vi "RT.Stages.Find.vi"(8 "Current Data":dbl[](array[numeric]), 9 "Voltage Data":dbl[](array[numeric]), 10 "Shots":T1[](array[typedef]) {"Results"."Off-Stage Min Volt" format="%#.6g"; "Results"."Off-Stage Avg Volt" format="%#.6g"; "Results"."Off-Stage Max Volt" format="%#.6g"; "Results"."Total Stage Time (us)" format="%#.6g"; "Results"."Off-Stage Avg Current" format="%#.6g"; "Results"."Total Voltage Pulses" format="%#.6g"; "Results"."Off-Stage Min Current" format="%#.6g"; "Results"."Off-Stage Max Current" format="%#.6g"}, 11 "Parameters":T3={"Shots"=0, "Shot.InitialVoltage"=0.0, "Shot.Stages"=0, "Stages"=[{"Stage.Dwell.Level"=0.0, "PullIn.Type"=enum."Pull In Transition Pulses", "PullIn.Level"=0.0, "Transition.Type"=enum."Stage Transition Voltage Increase", "Transition.Level"=0.0, "Results"={"Pull In Time"=TRUE, "Pull In Max Current"=TRUE, "Pull In Max Voltage"=TRUE, "Pull In Min Voltage"=TRUE, "Pull In Avg Voltage"=TRUE, "Hold Time"=TRUE, "Hold Max Current"=TRUE, "Hold Min Current"=TRUE, "Hold Avg Current"=TRUE, "Hold Max Voltage"=TRUE, "Hold Min Voltage"=TRUE, "Hold Avg Max Voltage"=TRUE, "Hold Avg Min Voltage"=TRUE, "Off Time"=TRUE, "Off Max Current"=TRUE, "Off Min Current"=TRUE, "Off Avg Current"=TRUE, "Off Max Voltage"=TRUE, "Off Min Voltage"=TRUE, "Off Avg Voltage"=TRUE, "Total Voltage Pulses"=TRUE, "Total Stage Time"=TRUE}}], "Timeout"=0.0, "Results.Count"=0, "Active Edge"=FALSE, "Rate.Hz"=0, "Channels"=0}) -> (2 "Shots":T1[](array[typedef]) {"Results"."Off-Stage Min Volt" format="%#.6g"; "Results"."Off-Stage Avg Volt" format="%#.6g"; "Results"."Off-Stage Max Volt" format="%#.6g"; "Results"."Total Stage Time (us)" format="%#.6g"; "Results"."Off-Stage Avg Current" format="%#.6g"; "Results"."Total Voltage Pulses" format="%#.6g"; "Results"."Off-Stage Min Current" format="%#.6g"; "Results"."Off-Stage Max Current" format="%#.6g"})   [LabVIEW 2019, in "Fuel Injector Analysis Addon Engine.lvlib"]
uses:
  Fuel Injector Analysis Addon Engine.lvlib
  Addon Shared/Types/Shot.Parameters.ctl
  Addon Shared/Types/Stage.Parameters.ctl
  Addon Shared/Types/Stage.PullIn.Types.ctl
  Addon Shared/Types/Stage.Transition.Types.ctl
  Addon Shared/Types/Analysis.Channels.Select.ctl
  RT Analysis/Controls/Shot Information Control.ctl
  Types/Stage.Measurements.ctl
  Types/Search.StateVariables.ctl
  Addon Shared/Types/Stage.Events.ctl
  Addon Shared/Fuel Injector Analysis Addon Shared.lvlib
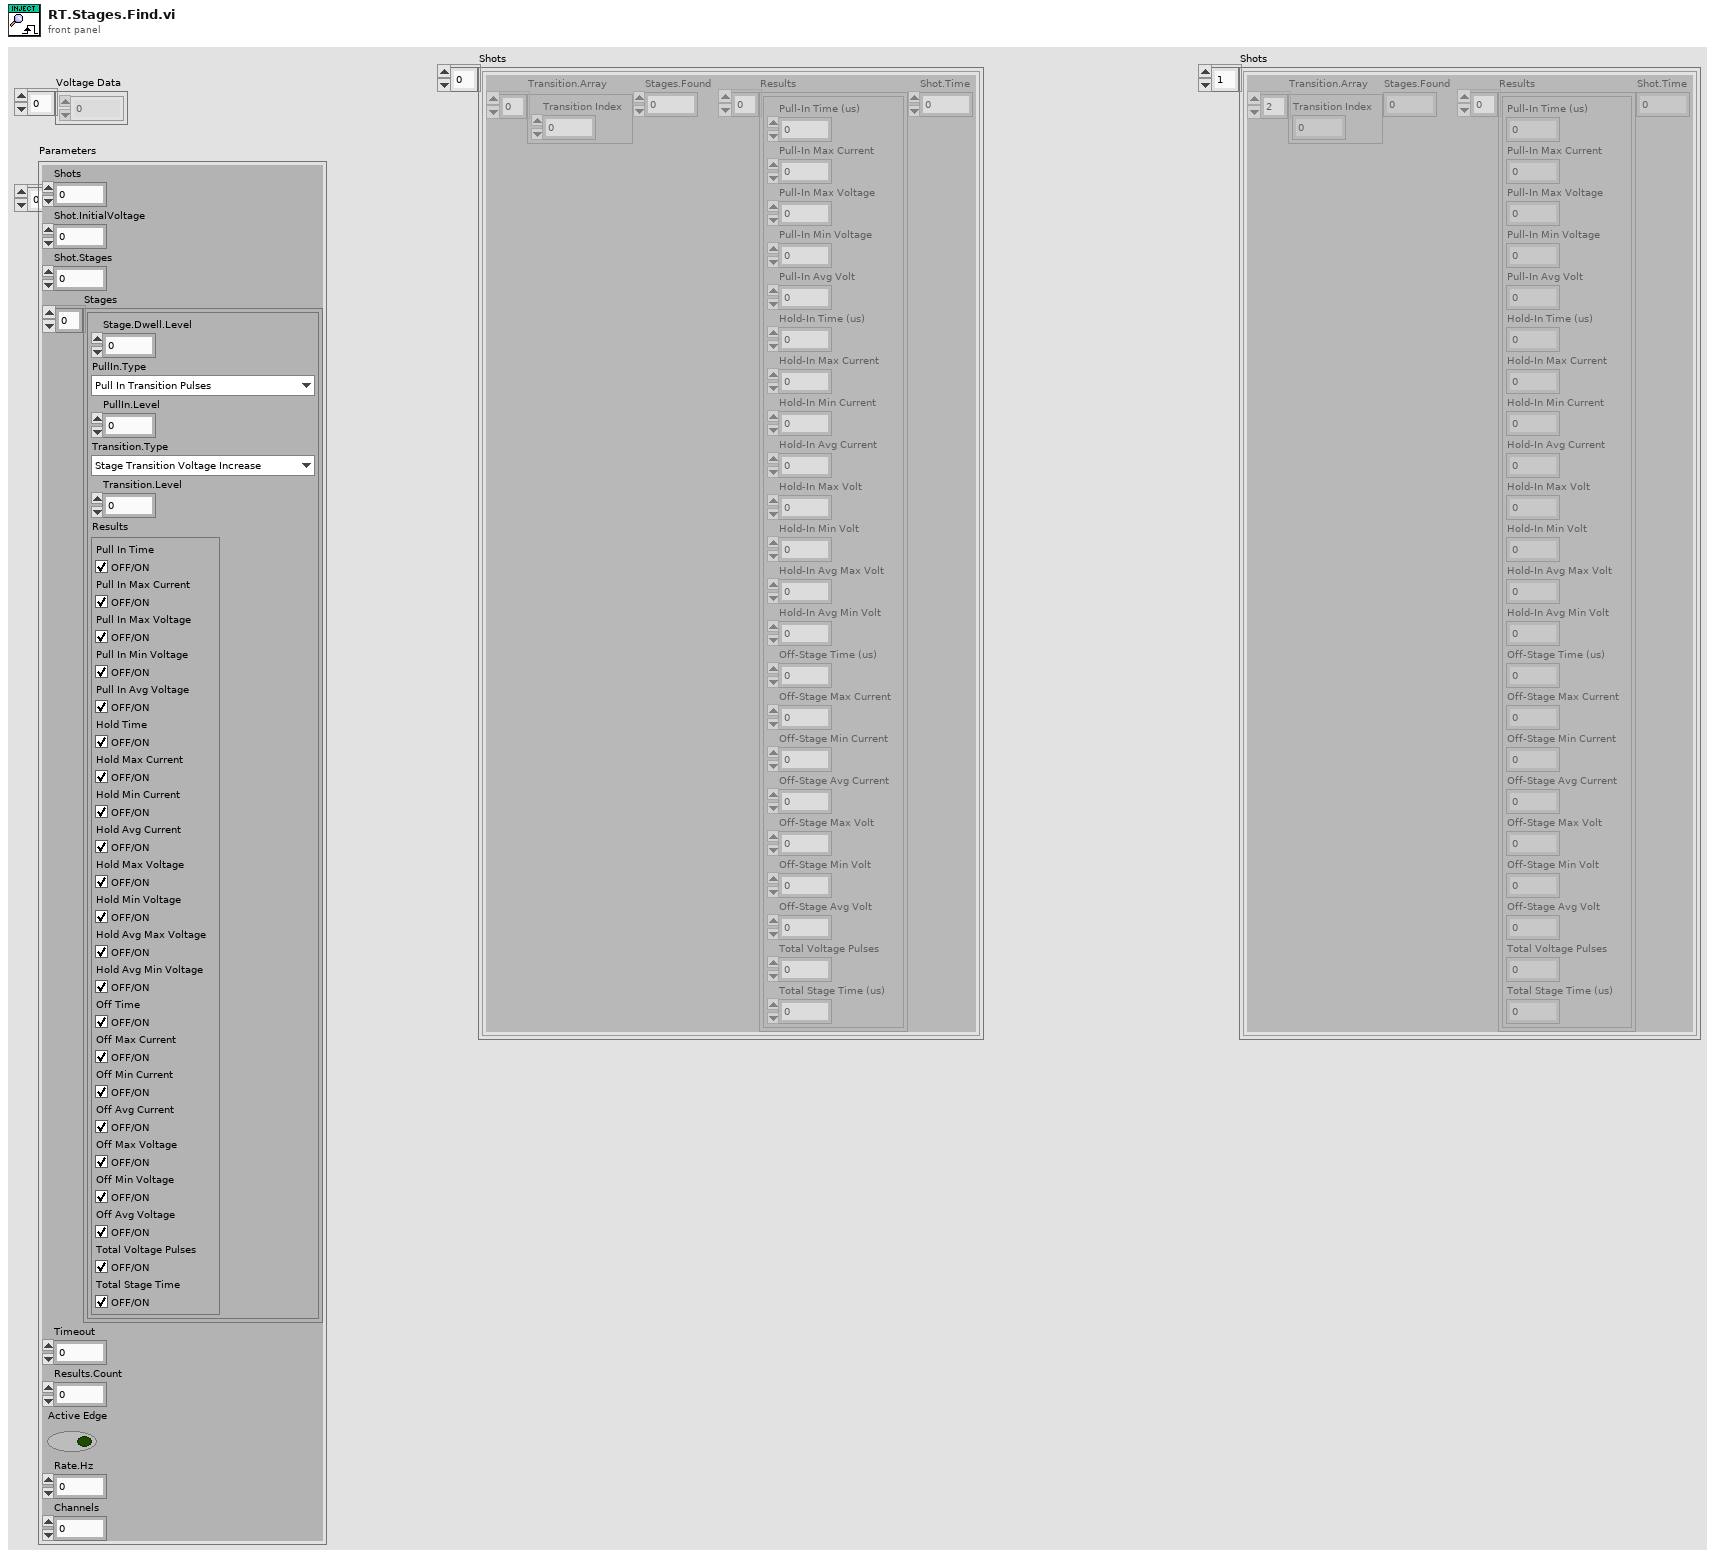
[diagram p1: front panel]
types:
  T1 = typedef "Fuel Injector Analysis Addon Engine.lvlib/Shot Information Control.ctl" = cluster{"Transition.Array":i32[], "Stages.Found":u16, "Results":T2[], "Shot.Time":dbl}
  T2 = typedef "Fuel Injector Analysis Addon Engine.lvlib/Stage.Measurements.ctl" = cluster{"Pull-In Time (us)":dbl, "Pull-In Max Current":dbl, "Pull-In Max Voltage":dbl, "Pull-In Min Voltage":dbl, "Pull-In Avg Volt":dbl, "Hold-In Time (us)":dbl, "Hold-In Max Current":dbl, "Hold-In Min Current":dbl, "Hold-In Avg Current":dbl, "Hold-In Max Volt":dbl, "Hold-In Min Volt":dbl, "Hold-In Avg Max Volt":dbl, "Hold-In Avg Min Volt":dbl, "Off-Stage Time (us)":dbl, "Off-Stage Max Current":dbl, "Off-Stage Min Current":dbl, "Off-Stage Avg Current":dbl, "Off-Stage Max Volt":dbl, "Off-Stage Min Volt":dbl, "Off-Stage Avg Volt":dbl, "Total Voltage Pulses":dbl, "Total Stage Time (us)":dbl}
  T3 = typedef "Fuel Injector Analysis Addon Shared.lvlib/Shot.Parameters.ctl" = cluster{"Shots":u32, "Shot.InitialVoltage":dbl, "Shot.Stages":u32, "Stages":T4[], "Timeout":dbl, "Results.Count":i32, "Active Edge":bool, "Rate.Hz":u32, "Channels":u32}
  T4 = typedef "Fuel Injector Analysis Addon Shared.lvlib/Stage.Parameters.ctl" = cluster{"Stage.Dwell.Level":dbl, "PullIn.Type":T5, "PullIn.Level":dbl, "Transition.Type":T6, "Transition.Level":dbl, "Results":T7}
  T5 = typedef "Fuel Injector Analysis Addon Shared.lvlib/Stage.PullIn.Types.ctl" = enum8{"Pull In Transition Pulses", "Pull In Transition Current Drop"}
  T6 = typedef "Fuel Injector Analysis Addon Shared.lvlib/Stage.Transition.Types.ctl" = enum8{"Stage Transition Inactive Time", "Stage Transition Voltage Increase", "Stage Transition Current Decrease", "Stage Transition Active Time"}
  T7 = typedef "Fuel Injector Analysis Addon Shared.lvlib/Analysis.Channels.Select.ctl" = cluster{"Pull In Time":bool, "Pull In Max Current":bool, "Pull In Max Voltage":bool, "Pull In Min Voltage":bool, "Pull In Avg Voltage":bool, "Hold Time":bool, "Hold Max Current":bool, "Hold Min Current":bool, "Hold Avg Current":bool, "Hold Max Voltage":bool, "Hold Min Voltage":bool, "Hold Avg Max Voltage":bool, "Hold Avg Min Voltage":bool, "Off Time":bool, "Off Max Current":bool, "Off Min Current":bool, "Off Avg Current":bool, "Off Max Voltage":bool, "Off Min Voltage":bool, "Off Avg Voltage":bool, "Total Voltage Pulses":bool, "Total Stage Time":bool}
  T8 = typedef "Fuel Injector Analysis Addon Engine.lvlib/Search.StateVariables.ctl" = cluster{"Dwell.Counts":i32, "Current.Max":dbl, "Stage.Index":i32, "Transition.Index":i32, "Transition":T9}
  T9 = typedef "Fuel Injector Analysis Addon Shared.lvlib/Stage.Events.ctl" = enum8{"PullIn.Start", "PullIn.End", "Dwell.End"}
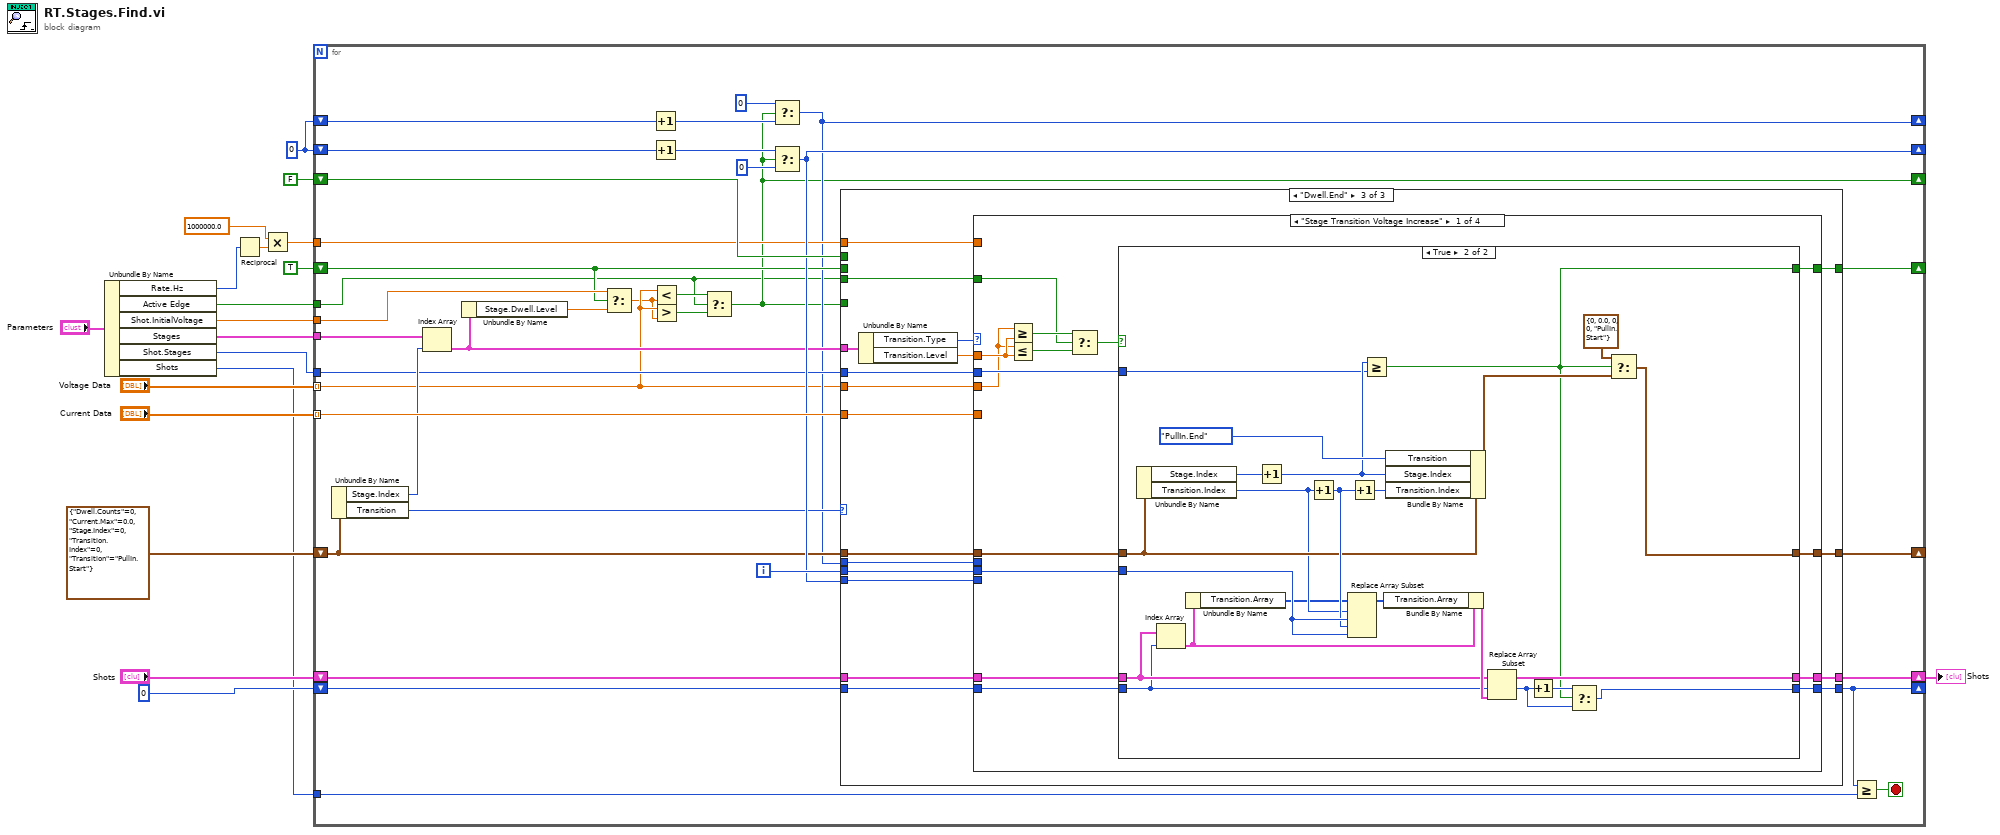
[diagram p0: block diagram]
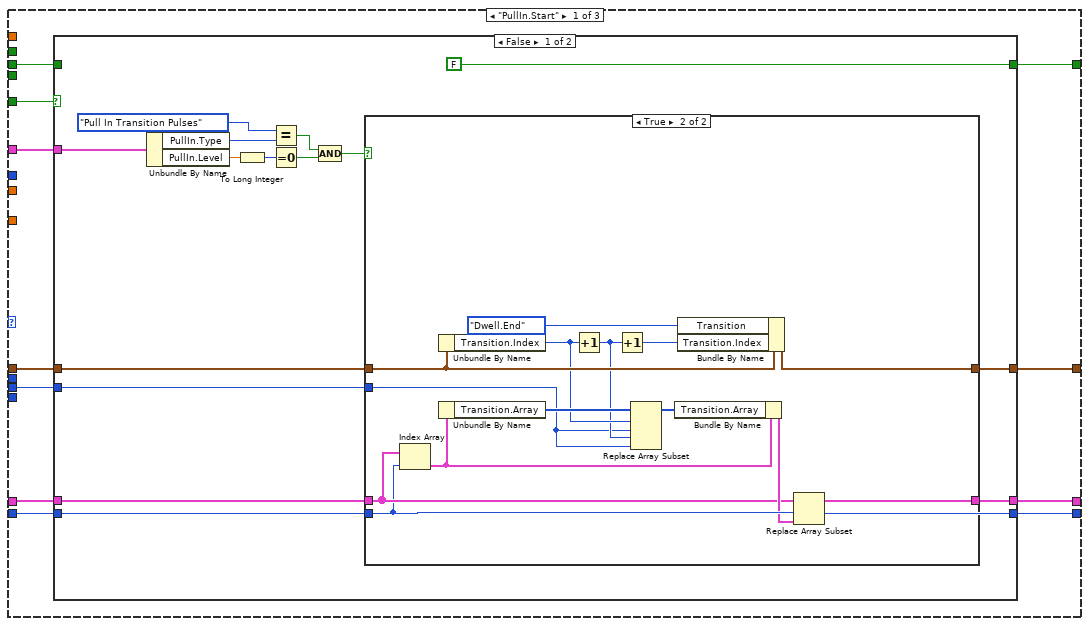
[diagram p2: hidden frame]
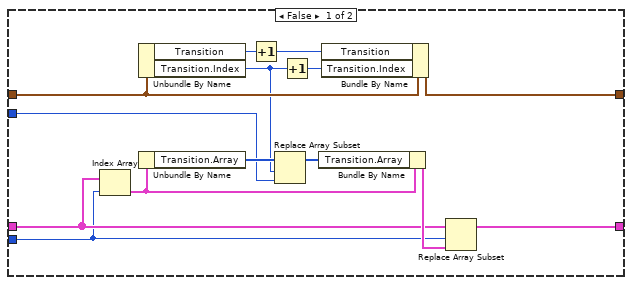
[diagram p3: hidden frame]
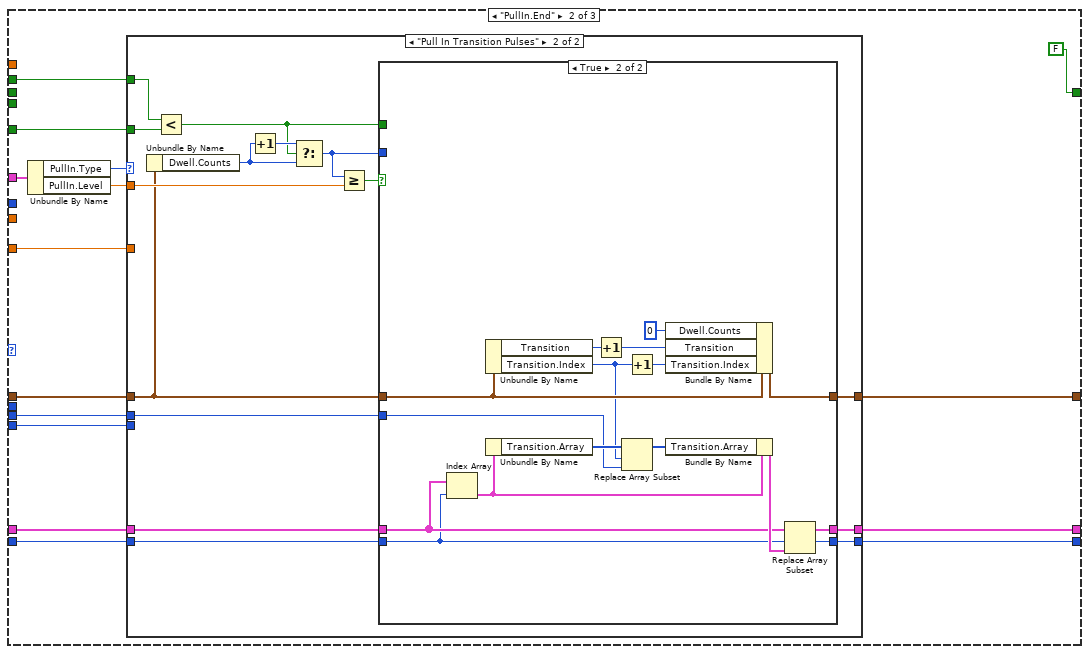
[diagram p5: hidden frame]
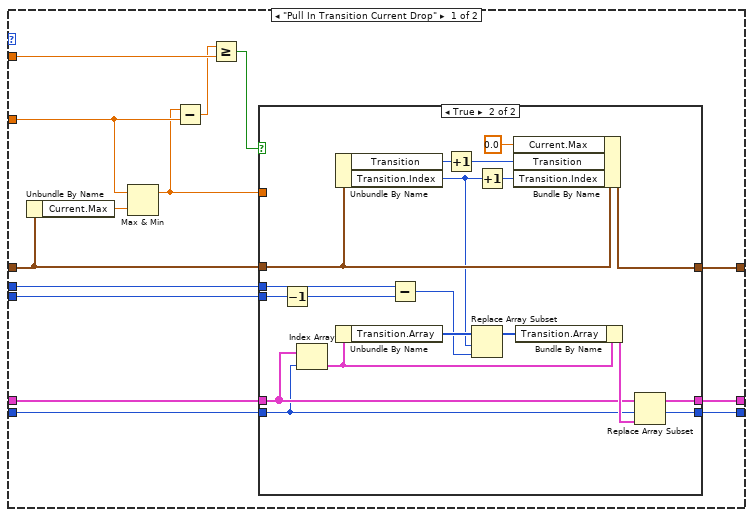
[diagram p6: hidden frame]
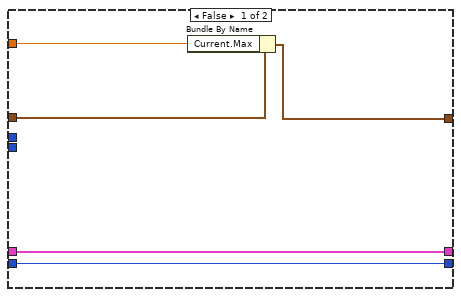
[diagram p7: hidden frame]
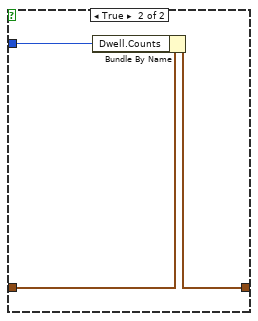
[diagram p9: hidden frame]
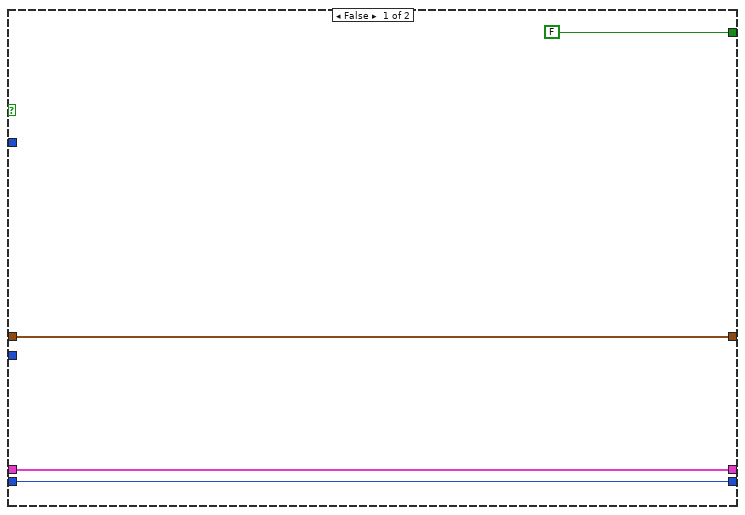
[diagram p10: hidden frame]
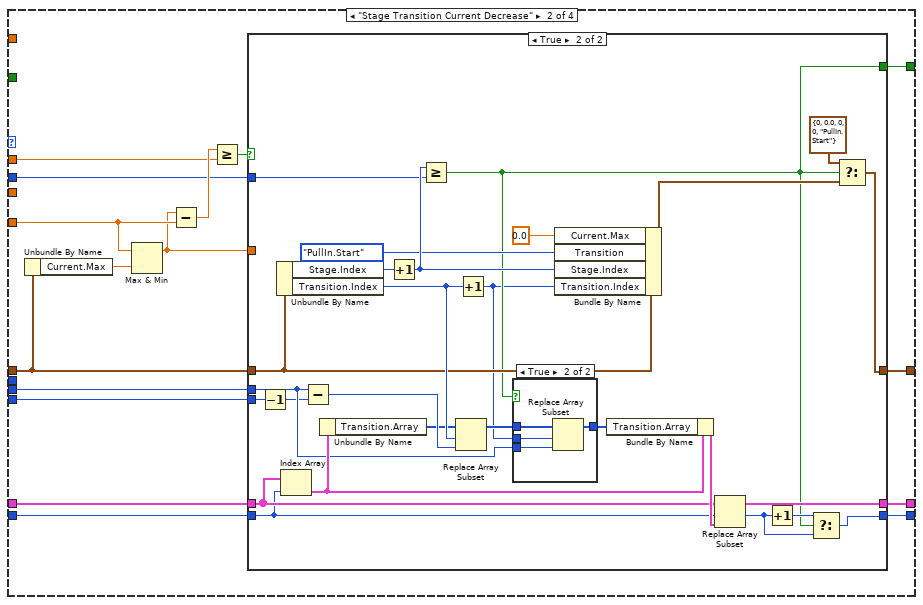
[diagram p11: hidden frame]
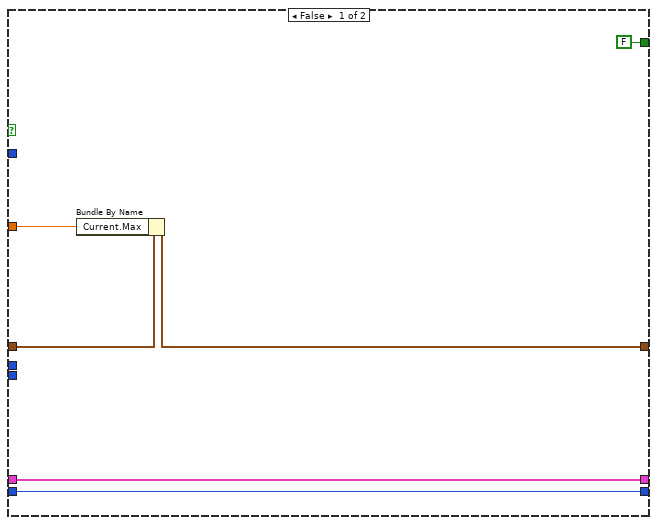
[diagram p12: hidden frame]
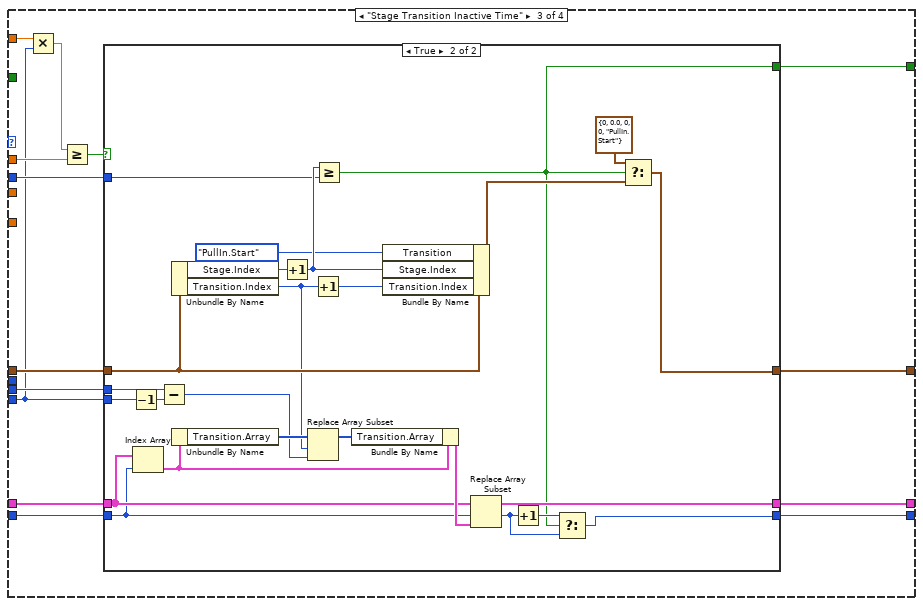
[diagram p14: hidden frame]
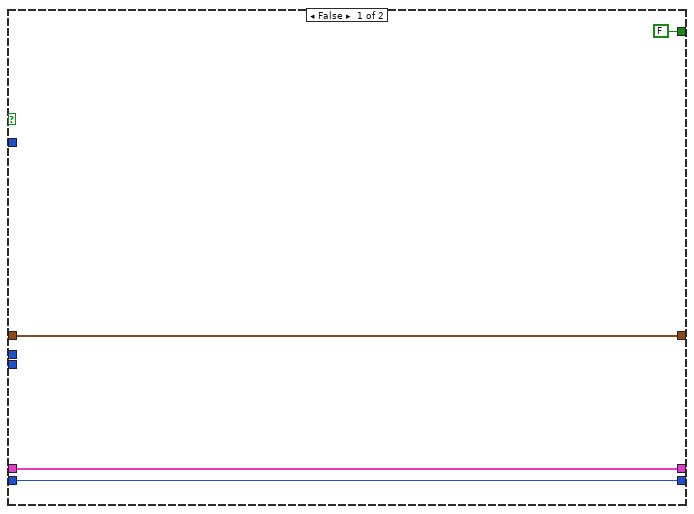
[diagram p15: hidden frame]
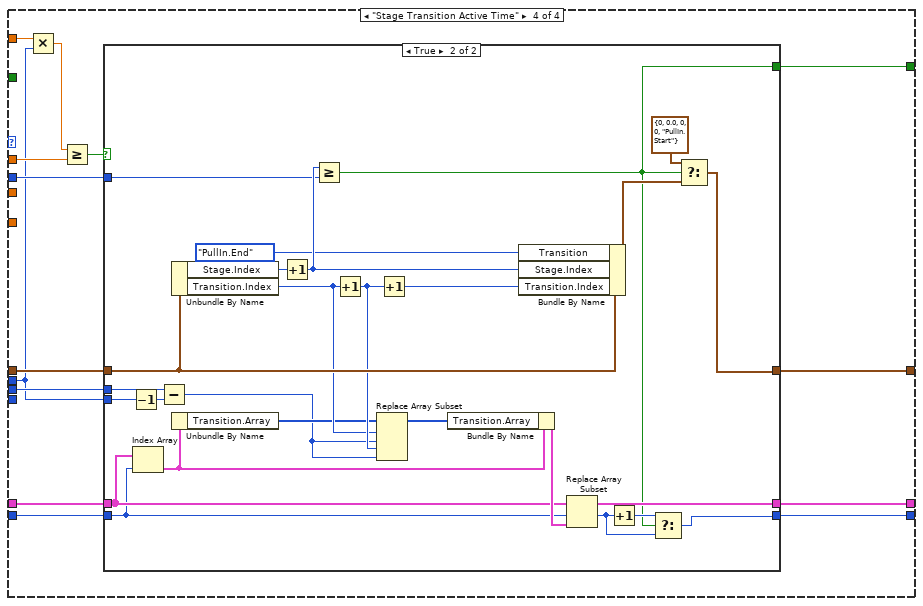
[diagram p16: hidden frame]
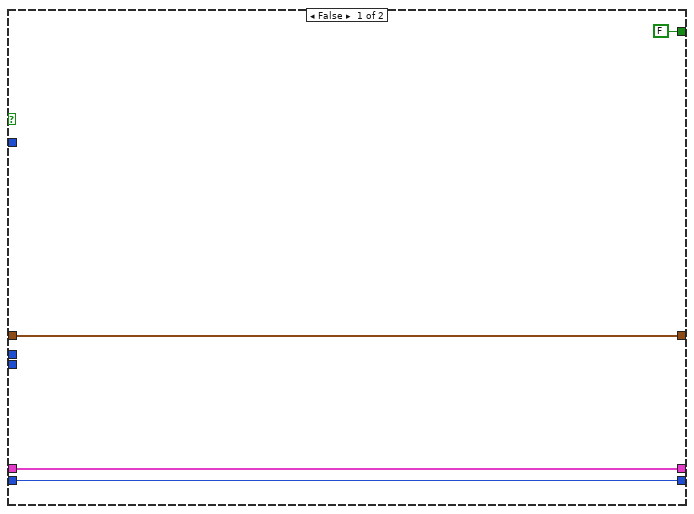
[diagram p17: hidden frame]
diagram:
  w3 = 0
  n1 = Unbundle By Name("Parameters") -> ("Rate.Hz"=w1:u32, "Active Edge"=w2:bool, "Shot.InitialVoltage"=w14:dbl, "Stages"=w15:T4[], "Shot.Stages"=w10:u32, "Shots"=w8:u32)
  n2 = Reciprocal(x=w1) -> (1/x=w6:dbl)
  n3 = Multiply(x=1000000.0, y=w6) -> (x*y=w5:dbl)
  n4 = for {
    tunnel: "Voltage Data" -> [w25] mode=indexing
    tunnel: "Current Data" -> [w53] mode=indexing
    tunnel: w15 -> [w54]
    shift-right: [w21] -> _
    shift-left: FALSE -> [w48]
    shift-right: [w47] -> _
    shift-left: w3 -> [w49]
    shift-right: [w42] -> _
    shift-left: T8 {"Dwell.Counts"=0, "Current.Max"=0.0, "Stage.Index"=0, "Transition.Index"=0, "Transition"=enum."PullIn.Start"} -> [w43]
    tunnel: w14 -> [w34]
    shift-right: [w40] -> w12
    shift-left: "Shots" -> [w41]
    shift-right: [w37] -> _
    shift-left: 0 -> [w39]
    tunnel: w10 -> [w38]
    tunnel: w8 -> [w36]
    shift-right: [w32] -> _
    shift-left: TRUE -> [w31]
    tunnel: w5 -> [w30]
    shift-right: [w26] -> _
    shift-left: w3 -> [w29]
    tunnel: w2 -> [w20]
    i -> [w52]
    stop <- w35 stop-if-true
    n5 = Unbundle By Name(w43) -> ("Stage.Index"=w44:i32, "Transition"=w45:T9)
    n6 = Index Array(array=w54, index=w44) -> (element=w46:T4)
    n7 = Unbundle By Name(w46) -> ("Stage.Dwell.Level"=w33:dbl)
    n8 = Select(t=w34, s=w31, f=w33) -> (s? t:f=w24:dbl)
    n9 = Increment(x=w29) -> (x+1=w28:i32)
    n10 = Increment(x=w49) -> (x+1=w51:i32)
    n11 = Less?(x=w25, y=w24) -> (x < y?=w22:bool)
    n12 = Greater?(x=w25, y=w24) -> (0:w23:bool)
    n13 = Select(t=w22, s=w20, f=w23) -> (s? t:f=w21:bool)
    n14 = Select(t=0 ("f"), s=w21, f=w28) -> (s? t:f=w26:i32)
    n15 = Select(t=w51, s=w21, f=0) -> (s? t:f=w47:i32)
    n16 = case shown="\"Dwell.End\"" w45 {
      tunnel: w53 -> [_ w127 w216]
      tunnel: w25 -> [_ _ w222]
      tunnel: w52 -> [w65 w124 w221]
      tunnel: w48 -> [_ w120 _]
      tunnel: w21 -> [w58 w121 _]
      tunnel: w47 -> [_ w123 w220]
      tunnel: w46 -> [w55 w126 w219]
      tunnel: w43 -> [w64 w119 w215]
      tunnel: [w63 w118 w214] -> w42
      tunnel: w41 -> [w62 w117 w213]
      tunnel: [w61 w114 w212] -> w40
      tunnel: w39 -> [w60 w116 w211]
      tunnel: [w59 w115 w210] -> w37
      tunnel: w38 -> [_ _ w209]
      tunnel: [w57 FALSE w208] -> w32
      tunnel: w31 -> [w56 _ _]
      tunnel: w30 -> [_ _ w207]
      tunnel: w26 -> [_ _ w206]
      tunnel: w20 -> [_ _ w205]
      frame "PullIn.Start" {
        n17 = case shown="False" w58 {
          tunnel: w65 -> [w76 _]
          tunnel: w64 -> [w80 w112]
          tunnel: [w79 w112] -> w63
          tunnel: w62 -> [w78 w111]
          tunnel: [w77 w111] -> w61
          tunnel: w60 -> [w75 w110]
          tunnel: [w75 w110] -> w59
          tunnel: [FALSE w109] -> w57
          tunnel: w56 -> [_ w109]
          tunnel: w55 -> [w73 _]
          frame False {
            n18 = Unbundle By Name(w73) -> ("PullIn.Type"=w72:T5, "PullIn.Level"=w70:dbl)
            n19 = To Long Integer(number=w70) -> (32bit integer=w69:i32)
            n20 = Equal?(x=Stage.PullIn.Types."Pull In Transition Pulses", y=w72) -> (x = y?=w68:bool)
            n21 = Equal To 0?(x=w69) -> (x = 0?=w67:bool)
            n22 = Compound Arithmetic op=AND(w68, w67) -> (w66:bool)
            n23 = case shown="True" w66 {
              tunnel: w80 -> [w93 w108]
              tunnel: [w90 w107] -> w79
              tunnel: w78 -> [w85 w102]
              tunnel: [w84 w101] -> w77
              tunnel: w76 -> [w83 w95]
              tunnel: w75 -> [w81 w99]
              frame False {
                n24 = Index Array(array=w85, index=w81) -> (element=w87:T1)
                n25 = Unbundle By Name(w93) -> ("Transition"=w94:T9, "Transition.Index"=w82:i32)
                n26 = Unbundle By Name(w87) -> ("Transition.Array"=w86:i32[])
                n27 = Increment(x=w94) -> (x+1=w91:T9)
                n28 = Replace Array Subset(array=w86, new element=w83, index=w82) -> (w89:i32[])
                n29 = Increment(x=w82) -> (x+1=w92:i32)
                n30 = Bundle By Name(cluster=w87, "Transition.Array"=w89) -> (w88:T1)
                n31 = Bundle By Name(cluster=w93, "Transition"=w91, "Transition.Index"=w92) -> (w90:T8)
                n32 = Replace Array Subset(array=w85, new element=w88, index=w81) -> (w84:T1[])
              }
              frame True {
                n33 = Index Array(array=w102, index=w99) -> (element=w104:T1)
                n34 = Unbundle By Name(w108) -> ("Transition.Index"=w100:i32)
                n35 = Unbundle By Name(w104) -> ("Transition.Array"=w103:i32[])
                n36 = Increment(x=w100) -> (x+1=w96:i32)
                n37 = Increment(x=w96) -> (x+1=w97:i32)
                n38 = Replace Array Subset(array=w103, new element #1=w95, index #1=w100, new element #2=w95, index #2=w96) -> (w106:i32[])
                n39 = Bundle By Name(cluster=w104, "Transition.Array"=w106) -> (w105:T1)
                n40 = Bundle By Name(cluster=w108, "Transition"=Stage.Events."Dwell.End", "Transition.Index"=w97) -> (w107:T8)
                n41 = Replace Array Subset(array=w102, new element=w105, index=w99) -> (w101:T1[])
              }
            }
          }
          frame True {
          }
        }
      }
      frame "PullIn.End" {
        n42 = Unbundle By Name(w126) -> ("PullIn.Type"=w122:T5, "PullIn.Level"=w125:dbl)
        n43 = case shown="\"Pull In Transition Pulses\"" w122 {
          tunnel: w127 -> [w141 _]
          tunnel: w125 -> [w140 w179]
          tunnel: w124 -> [w138 w173]
          tunnel: w123 -> [w137 _]
          tunnel: w121 -> [_ w176]
          tunnel: w120 -> [_ w175]
          tunnel: w119 -> [w134 w172]
          tunnel: [w132 w174] -> w118
          tunnel: w117 -> [w131 w168]
          tunnel: w116 -> [w130 w167]
          tunnel: [w129 w166] -> w115
          tunnel: [w128 w165] -> w114
          frame "Pull In Transition Current Drop" {
            n44 = Unbundle By Name(w134) -> ("Current.Max"=w135:dbl)
            n45 = Max & Min(x=w141, y=w135) -> (max(x,y)=w133:dbl)  [unwired: 1 out]
            n46 = Subtract(x=w133, y=w141) -> (x-y=w136:dbl)
            n47 = Greater Or Equal?(x=w136, y=w140) -> (x >= y?=w139:bool)
            n48 = case shown="True" w139 {
              tunnel: w138 -> [_ w164]
              tunnel: w137 -> [_ w163]
              tunnel: w134 -> [w146 w157]
              tunnel: w133 -> [w145 _]
              tunnel: [w144 w158] -> w132
              tunnel: w131 -> [w142 w152]
              tunnel: w130 -> [w143 w149]
              tunnel: [w143 w149] -> w129
              tunnel: [w142 w148] -> w128
              frame False {
                n49 = Bundle By Name(cluster=w146, "Current.Max"=w145) -> (w144:T8)
              }
              frame True {
                n50 = Decrement(x=w163) -> (x-1=w147:i32)
                n51 = Index Array(array=w152, index=w149) -> (element=w154:T1)
                n52 = Unbundle By Name(w157) -> ("Transition"=w159:T9, "Transition.Index"=w150:i32)
                n53 = Unbundle By Name(w154) -> ("Transition.Array"=w153:i32[])
                n54 = Subtract(x=w164, y=w147) -> (x-y=w151:i32)
                n55 = Increment(x=w159) -> (x+1=w161:T9)
                n56 = Replace Array Subset(array=w153, new element=w151, index=w150) -> (w156:i32[])
                n57 = Increment(x=w150) -> (x+1=w160:i32)
                n58 = Bundle By Name(cluster=w157, "Current.Max"=0.0 ("Dwell.Counts"), "Transition"=w161, "Transition.Index"=w160) -> (w158:T8)
                n59 = Bundle By Name(cluster=w154, "Transition.Array"=w156) -> (w155:T1)
                n60 = Replace Array Subset(array=w152, new element=w155, index=w149) -> (w148:T1[])
              }
            }
          }
          frame "Pull In Transition Pulses" {
            n61 = Unbundle By Name(w172) -> ("Dwell.Counts"=w171:i32)
            n62 = Less?(x=w175, y=w176) -> (x < y?=w169:bool)
            n63 = Increment(x=w171) -> (x+1=w177:i32)
            n64 = Select(t=w177, s=w169, f=w171) -> (s? t:f=w170:i32)
            n65 = Greater Or Equal?(x=w170, y=w179) -> (x >= y?=w178:bool)
            n66 = case shown="True" w178 {
              tunnel: w172 -> [w185 w201]
              tunnel: [w184 w200] -> w174
              tunnel: w173 -> [_ w192]
              tunnel: w170 -> [w183 _]
              tunnel: w169 -> [w182 _]
              tunnel: w168 -> [w180 w194]
              tunnel: w167 -> [w181 w193]
              tunnel: [w181 w193] -> w166
              tunnel: [w180 w190] -> w165
              frame False {
                n67 = case shown="False" w182 {
                  tunnel: w185 -> [w186 w189]
                  tunnel: [w186 w188] -> w184
                  tunnel: w183 -> [_ w187]
                  frame False {
                  }
                  frame True {
                    n68 = Bundle By Name(cluster=w189, "Dwell.Counts"=w187) -> (w188:T8)
                  }
                }
              }
              frame True {
                n69 = Index Array(array=w194, index=w193) -> (element=w196:T1)
                n70 = Unbundle By Name(w201) -> ("Transition"=w204:T9, "Transition.Index"=w191:i32)
                n71 = Unbundle By Name(w196) -> ("Transition.Array"=w195:i32[])
                n72 = Increment(x=w204) -> (x+1=w202:T9)
                n73 = Replace Array Subset(array=w195, new element=w192, index=w191) -> (w198:i32[])
                n74 = Increment(x=w191) -> (x+1=w203:i32)
                n75 = Bundle By Name(cluster=w201, "Dwell.Counts"=0, "Transition"=w202, "Transition.Index"=w203) -> (w200:T8)
                n76 = Bundle By Name(cluster=w196, "Transition.Array"=w198) -> (w197:T1)
                n77 = Replace Array Subset(array=w194, new element=w197, index=w193) -> (w190:T1[])
              }
            }
          }
        }
      }
      frame "Dwell.End" {
        n78 = Unbundle By Name(w219) -> ("Transition.Type"=w218:T6, "Transition.Level"=w217:dbl)
        n79 = case shown="\"Stage Transition Voltage Increase\"" w218 {
          tunnel: w222 -> [w227 _ _ _]
          tunnel: w221 -> [w237 w275 w327 w369]
          tunnel: w217 -> [w228 w277 w329 w371]
          tunnel: w220 -> [_ w274 w319 _]
          tunnel: w216 -> [_ w278 _ _]
          tunnel: w215 -> [w236 w273 w328 w370]
          tunnel: [w235 w271 w326 w368] -> w214
          tunnel: w213 -> [w234 w269 w325 w367]
          tunnel: [w233 w268 w323 w365] -> w212
          tunnel: w211 -> [w232 w267 w324 w366]
          tunnel: [w231 w266 w322 w364] -> w210
          tunnel: w209 -> [w230 w265 w321 w363]
          tunnel: [w229 w264 w320 w362] -> w208
          tunnel: w207 -> [_ _ w318 w361]
          tunnel: w206 -> [_ _ _ w359]
          tunnel: w205 -> [w223 _ _ _]
          frame "Stage Transition Voltage Increase" {
            n80 = Greater Or Equal?(x=w227, y=w228) -> (x >= y?=w225:bool)
            n81 = Less Or Equal?(x=w227, y=w228) -> (x <= y?=w226:bool)
            n82 = Select(t=w225, s=w223, f=w226) -> (s? t:f=w224:bool)
            n83 = case shown="True" w224 {
              tunnel: w237 -> [_ w263]
              tunnel: w236 -> [w241 w258]
              tunnel: [w241 w245] -> w235
              tunnel: w234 -> [w240 w253]
              tunnel: [w240 w252] -> w233
              tunnel: w232 -> [w239 w243]
              tunnel: [w239 w244] -> w231
              tunnel: w230 -> [_ w247]
              tunnel: [FALSE w242] -> w229
              frame False {
              }
              frame True {
                n84 = Unbundle By Name(w258) -> ("Stage.Index"=w259:i32, "Transition.Index"=w257:i32)
                n85 = Index Array(array=w253, index=w243) -> (element=w254:T1)
                n86 = Unbundle By Name(w254) -> ("Transition.Array"=w251:i32[])
                n87 = Increment(x=w259) -> (x+1=w260:i32)
                n88 = Increment(x=w257) -> (x+1=w262:i32)
                n89 = Replace Array Subset(array=w251, new element #1=w263, index #1=w257, new element #2=w263, index #2=w262) -> (w250:i32[])
                n90 = Increment(x=w262) -> (x+1=w256:i32)
                n91 = Greater Or Equal?(x=w260, y=w247) -> (x >= y?=w242:bool)
                n92 = Bundle By Name(cluster=w254, "Transition.Array"=w250) -> (w255:T1)
                n93 = Bundle By Name(cluster=w258, "Transition"=Stage.Events."PullIn.End" ("PullIn.Type"), "Stage.Index"=w260, "Transition.Index"=w256) -> (w246:T8)
                n94 = Replace Array Subset(array=w253, new element=w255, index=w243) -> (w252:T1[])
                n95 = Increment(x=w243) -> (x+1=w249:i32)
                n96 = Select(t=w249, s=w242, f=w243) -> (s? t:f=w244:i32)
                n97 = Select(t=T8 {"Dwell.Counts"=0, "Current.Max"=0.0, "Stage.Index"=0, "Transition.Index"=0, "Transition"=enum."PullIn.Start"}, s=w242, f=w246) -> (s? t:f=w245:T8)
              }
            }
          }
          frame "Stage Transition Current Decrease" {
            n98 = Unbundle By Name(w273) -> ("Current.Max"=w272:dbl)
            n99 = Max & Min(x=w278, y=w272) -> (max(x,y)=w270:dbl)  [unwired: 1 out]
            n100 = Subtract(x=w270, y=w278) -> (x-y=w279:dbl)
            n101 = Greater Or Equal?(x=w279, y=w277) -> (x >= y?=w276:bool)
            n102 = case shown="True" w276 {
              tunnel: w274 -> [_ w311]
              tunnel: w273 -> [w285 w309]
              tunnel: w275 -> [_ w287]
              tunnel: [w283 w296] -> w271
              tunnel: w270 -> [w284 _]
              tunnel: w269 -> [w282 w302]
              tunnel: [w282 w301] -> w268
              tunnel: w267 -> [w281 w294]
              tunnel: [w281 w293] -> w266
              tunnel: w265 -> [_ w298]
              tunnel: [FALSE w291] -> w264
              frame False {
                n103 = Bundle By Name(cluster=w285, "Current.Max"=w284) -> (w283:T8)
              }
              frame True {
                n104 = Decrement(x=w311) -> (x-1=w286:i32)
                n105 = Unbundle By Name(w309) -> ("Stage.Index"=w308:i32, "Transition.Index"=w310:i32)
                n106 = Index Array(array=w302, index=w294) -> (element=w300:T1)
                n107 = Subtract(x=w287, y=w286) -> (x-y=w305:i32)
                n108 = Unbundle By Name(w300) -> ("Transition.Array"=w299:i32[])
                n109 = Increment(x=w308) -> (x+1=w307:i32)
                n110 = Greater Or Equal?(x=w307, y=w298) -> (x >= y?=w291:bool)
                n111 = Replace Array Subset(array=w299, new element=w305, index=w310) -> (w290:i32[])
                n112 = Increment(x=w310) -> (x+1=w288:i32)
                n113 = case shown="True" w291 {
                  tunnel: w290 -> [w312 w316]
                  tunnel: [w312 w315] -> w289
                  tunnel: w288 -> [_ w314]
                  tunnel: w287 -> [_ w313]
                  frame False {
                  }
                  frame True {
                    n114 = Replace Array Subset(array=w316, new element=w313, index=w314) -> (w315:i32[])
                  }
                }
                n115 = Bundle By Name(cluster=w309, "Current.Max"=0.0, "Transition"=Stage.Events."PullIn.Start" ("PullIn.Type"), "Stage.Index"=w307, "Transition.Index"=w288) -> (w297:T8)
                n116 = Bundle By Name(cluster=w300, "Transition.Array"=w289) -> (w303:T1)
                n117 = Replace Array Subset(array=w302, new element=w303, index=w294) -> (w301:T1[])
                n118 = Increment(x=w294) -> (x+1=w295:i32)
                n119 = Select(t=w295, s=w291, f=w294) -> (s? t:f=w293:i32)
                n120 = Select(t=T8 {"Dwell.Counts"=0, "Current.Max"=0.0, "Stage.Index"=0, "Transition.Index"=0, "Transition"=enum."PullIn.Start"}, s=w291, f=w297) -> (s? t:f=w296:T8)
              }
            }
          }
          frame "Stage Transition Inactive Time" {
            n121 = Multiply(x=w318, y=w319) -> (x*y=w317:dbl)
            n122 = Greater Or Equal?(x=w317, y=w329) -> (x >= y?=w330:bool)
            n123 = case shown="True" w330 {
              tunnel: w319 -> [_ w358]
              tunnel: w328 -> [w334 w356]
              tunnel: w327 -> [_ w352]
              tunnel: [w334 w339] -> w326
              tunnel: w325 -> [w333 w347]
              tunnel: w324 -> [w332 w338]
              tunnel: [w333 w344] -> w323
              tunnel: [w332 w337] -> w322
              tunnel: w321 -> [_ w341]
              tunnel: [FALSE w336] -> w320
              frame False {
              }
              frame True {
                n124 = Decrement(x=w358) -> (x-1=w335:i32)
                n125 = Index Array(array=w347, index=w338) -> (element=w349:T1)
                n126 = Subtract(x=w352, y=w335) -> (x-y=w346:i32)
                n127 = Unbundle By Name(w356) -> ("Stage.Index"=w355:i32, "Transition.Index"=w345:i32)
                n128 = Unbundle By Name(w349) -> ("Transition.Array"=w348:i32[])
                n129 = Increment(x=w355) -> (x+1=w354:i32)
                n130 = Replace Array Subset(array=w348, new element=w346, index=w345) -> (w351:i32[])
                n131 = Increment(x=w345) -> (x+1=w357:i32)
                n132 = Greater Or Equal?(x=w354, y=w341) -> (x >= y?=w336:bool)
                n133 = Bundle By Name(cluster=w349, "Transition.Array"=w351) -> (w350:T1)
                n134 = Bundle By Name(cluster=w356, "Transition"=Stage.Events."PullIn.Start" ("PullIn.Type"), "Stage.Index"=w354, "Transition.Index"=w357) -> (w340:T8)
                n135 = Replace Array Subset(array=w347, new element=w350, index=w338) -> (w344:T1[])
                n136 = Increment(x=w338) -> (x+1=w343:i32)
                n137 = Select(t=w343, s=w336, f=w338) -> (s? t:f=w337:i32)
                n138 = Select(t=T8 {"Dwell.Counts"=0, "Current.Max"=0.0, "Stage.Index"=0, "Transition.Index"=0, "Transition"=enum."PullIn.Start"}, s=w336, f=w340) -> (s? t:f=w339:T8)
              }
            }
          }
          frame "Stage Transition Active Time" {
            n139 = Multiply(x=w361, y=w359) -> (x*y=w360:dbl)
            n140 = Greater Or Equal?(x=w360, y=w371) -> (x >= y?=w372:bool)
            n141 = case shown="True" w372 {
              tunnel: w359 -> [_ w401]
              tunnel: w370 -> [w376 w400]
              tunnel: w369 -> [_ w396]
              tunnel: [w376 w387] -> w368
              tunnel: w367 -> [w375 w393]
              tunnel: w366 -> [w374 w386]
              tunnel: [w375 w392] -> w365
              tunnel: [w374 w385] -> w364
              tunnel: w363 -> [_ w389]
              tunnel: [FALSE w384] -> w362
              frame False {
              }
              frame True {
                n142 = Decrement(x=w401) -> (x-1=w383:i32)
                n143 = Index Array(array=w393, index=w386) -> (element=w394:T1)
                n144 = Subtract(x=w396, y=w383) -> (x-y=w377:i32)
                n145 = Unbundle By Name(w400) -> ("Stage.Index"=w399:i32, "Transition.Index"=w381:i32)
                n146 = Unbundle By Name(w394) -> ("Transition.Array"=w379:i32[])
                n147 = Increment(x=w399) -> (x+1=w398:i32)
                n148 = Greater Or Equal?(x=w398, y=w389) -> (x >= y?=w384:bool)
                n149 = Increment(x=w381) -> (x+1=w382:i32)
                n150 = Replace Array Subset(array=w379, new element #1=w377, index #1=w381, new element #2=w377, index #2=w382) -> (w378:i32[])
                n151 = Increment(x=w382) -> (x+1=w380:i32)
                n152 = Bundle By Name(cluster=w394, "Transition.Array"=w378) -> (w395:T1)
                n153 = Bundle By Name(cluster=w400, "Transition"=Stage.Events."PullIn.End" ("PullIn.Type"), "Stage.Index"=w398, "Transition.Index"=w380) -> (w388:T8)
                n154 = Replace Array Subset(array=w393, new element=w395, index=w386) -> (w392:T1[])
                n155 = Increment(x=w386) -> (x+1=w391:i32)
                n156 = Select(t=w391, s=w384, f=w386) -> (s? t:f=w385:i32)
                n157 = Select(t=T8 {"Dwell.Counts"=0, "Current.Max"=0.0, "Stage.Index"=0, "Transition.Index"=0, "Transition"=enum."PullIn.Start"}, s=w384, f=w388) -> (s? t:f=w387:T8)
              }
            }
          }
        }
      }
    }
    n158 = Greater Or Equal?(x=w37, y=w36) -> (x >= y?=w35:bool)
  }
  "Shots" <- w12
